vi "merlinSetFrequency.vi"(8 "error in":errorcluster, 10 "Freq":u32, 11 "Port":refnum<visa-resource-name>) -> (0 "error out":errorcluster, 3 "Port out":refnum<visa-resource-name>)   [LabVIEW 2021]
panel:
  out "concatenated string":string
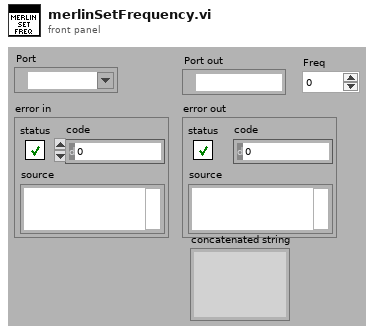
[diagram p1: front panel]
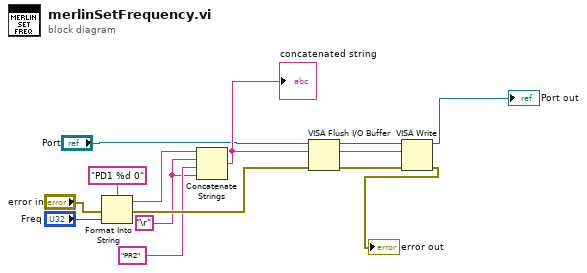
[diagram p0: block diagram]
diagram:
  w6 = "\r"
  n1 = Format Into String(format string="PD1 %d 0" ("concatenated string"), error in="error in", "Freq") -> (resulting string=w12:string, error out=w11:errorcluster)  [unwired: 1 in]
  n2 = Concatenate Strings(w12, w6, "PR2" ("concatenated string"), w6) -> (w8:string)
  "concatenated string" <- w8
  n3 = VISA Flush I/O Buffer(VISA resource name="Port", error in (no error)=w11) -> (VISA resource name out=w1:refnum<visa-resource-name>, error out=w3:errorcluster)  [unwired: 1 in]
  n4 = VISA Write(VISA resource name=w1, write buffer=w8, error in (no error)=w3) -> (VISA resource name out=→"Port out":refnum<visa-resource-name>, error out=→"error out":errorcluster)  [unwired: 1 out]
